vi "Constants.vi"() -> ()   [LabVIEW 2015, in "Development Tools Examples Shared.lvlib"]
doc: "Use this Global VI to access the GUIDs assigned to the page resources of the Custom Device."
uses:
  Development Tools Examples Shared.lvlib
panel:
  in  "Tab Control":enum32{"GUIDS", "Constants", "Properties"}(tab)
  in  "Extra5":string="d73f1a02-2631-461f-ab2a-6db747e9e32f"
  in  "Extra4":string="fb24e185-1071-4b44-a3a8-c31abe3238b8"
  in  "Extra3":string="fc0f4418-f86b-4d7f-bfba-57ff7a0fe79f"
  in  "Extra2":string="737ee67f-c0c4-40f9-9da4-7090f62c5999"
  in  "Extra1":string="ee00d7ec-8989-46a0-8cb1-5dba9537858e"
  in  "Custom Device XML Editor":string="1ca38015-fda9-4fcc-96bd-c39a2a0966e9"
  in  "Target Dependency Validation":string="236ba180-38b2-4067-b903-51e377536b9e"
  in  "Host Dependency Validation":string="99003fca-bc00-4e11-813a-550b118cc181"
  in  "Compatible Device Detection":string="3f10f15f-eaac-42d5-800e-6ed9a110e412"
  in  "Saving and Loading Configurations":string="f3dfc745-ee33-4d05-b2e4-57350711bddf"
  in  "Help Files":string="fdf68f10-9de1-44bc-8b47-931a3c579c52"
  in  "Errors":string="6b16e173-82d5-42e9-a892-d10f89a4f636"
  in  "Development Tools Examples":string="bfffa973-ae72-4159-bc33-e28886d74963"
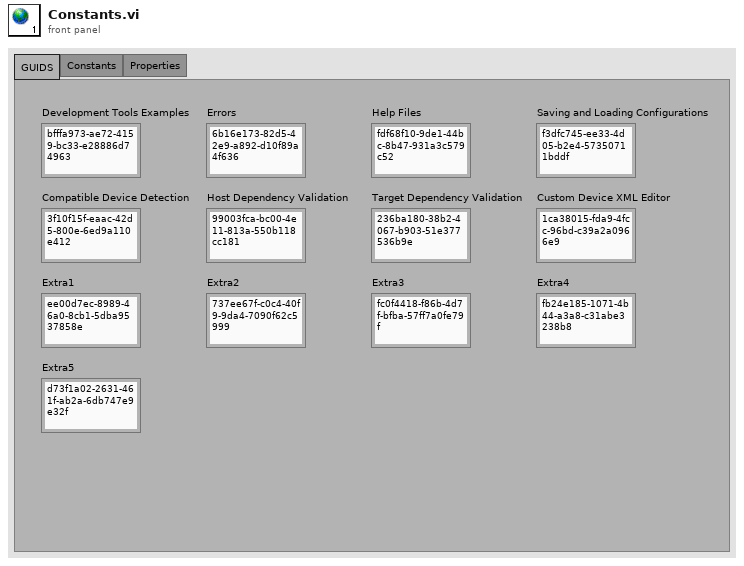
[diagram p1: front panel]
diagram:
